vi "Script MessageName.vi"(4 "Message Paths":T5, 6 "Message":T1, 7 "App":refnum<vi>, 8 "error in (no error)":errorcluster, 11 "LV-Protoc in":refnum<class "LV-Protoc.lvclass">) -> (0 "error out":errorcluster, 3 "LV-Protoc out":refnum<class "LV-Protoc.lvclass">)   [LabVIEW 2020, in "LV-Protoc.lvlib" / "LV-Protoc.lvclass"]
uses:
  LV-Protoc.lvclass
  Message Paths.ctl
  LV-Proto/Message.ctl
  LV-Proto/Field.ctl
  LV-Proto/Type.ctl
  LV-Proto/Proto Type.ctl
  <vilib>/Utility/traverseref.llb/TRef TravTarget.ctl
  LV-Protoc.lvlib
  LV-Proto/LV-Proto.lvlib
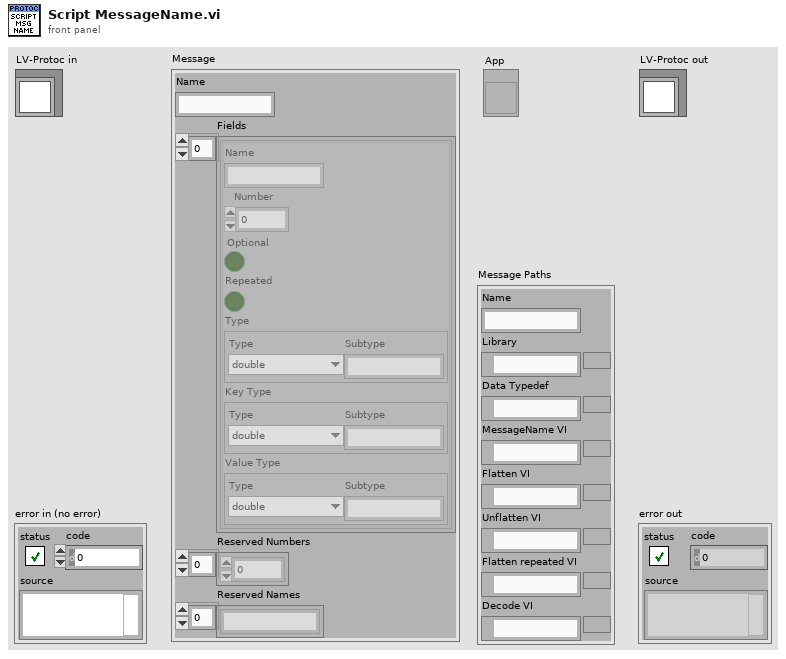
[diagram p1: front panel]
types:
  T1 = typedef "LV-Proto.lvlib/Message.ctl" = cluster{"Name":string, "Fields":T2[], "Reserved Numbers":u32[], "Reserved Names":string[]}
  T2 = typedef "LV-Proto.lvlib/Field.ctl" = cluster{"Name":string, "Number":u32, "Optional":bool, "Repeated":bool, "Type":T3, "Key Type":T3, "Value Type":T3}
  T3 = typedef "LV-Proto.lvlib/Type.ctl" = cluster{"Type":T4, "Subtype":string}
  T4 = typedef "LV-Proto.lvlib/Proto Type.ctl" = enum16{"UNKNOWN", "double", "float", "int32", "int64", "uint32", "uint64", "sint32", "sint64", "fixed32", "fixed64", "sfixed32", "sfixed64", "bool", "string", "bytes", "enum", "map", "message"}
  T5 = typedef "LV-Protoc.lvlib/Message Paths.ctl" = cluster{"Name":string, "Library":path, "Data Typedef":path, "MessageName VI":path, "Flatten VI":path, "Unflatten VI":path, "Flatten repeated VI":path, "Decode VI":path}
  T6 = typedef "TRef TravTarget.ctl" = enum16{"FP", "BD", "Other"}
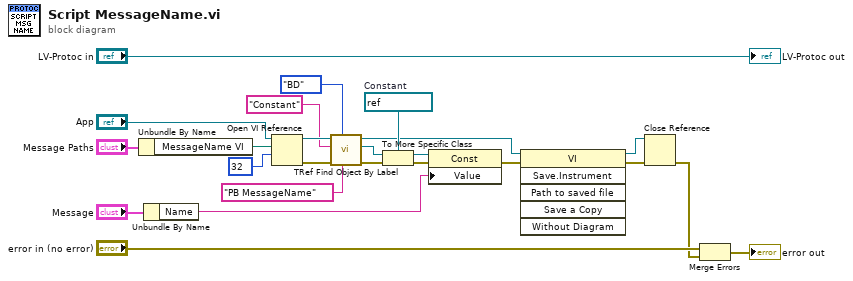
[diagram p0: block diagram]
diagram:
  w11 = refnum<vi> refnum  # Constant
  n1 = Unbundle By Name("Message Paths") -> ("MessageName VI"=w20:path)
  n2 = Unbundle By Name("Message") -> ("Name"=w8:string)
  n3 = Open VI Reference(application reference (local)="App", vi path=w20, options=32) -> (vi reference=w18:refnum<vi>, error out=w17:errorcluster)  [unwired: 3 in]
  n4 = call <vilib>:"TRef Find Object By Label.vi"("Label"="PB MessageName", "Traverse Target"=TRef_TravTarget."BD", "error in (no error)"=w17, "Class Name"="Constant", "VI Ref"=w18) -> ("error out"=w13:errorcluster, "Found Obj Ref"=w12:refnum<vi>, "dup VI Ref"=w5:refnum<vi>)  [unwired: 3 in, 1 out]
  n5 = To More Specific Class(target class=w11, reference=w12, error in=w13) -> (specific class reference=w9:refnum<vi>, error out=w10:errorcluster)
  n6 = property class="Const"(reference=w9, error in=w10, "Value"=w8) -> (error out=w6:errorcluster)  [unwired: 1 out]
  n7 = invoke class="VI" method="Save.Instrument"(reference=w5, error in=w6) -> (reference out=w3:refnum<vi>, error out=w4:errorcluster)  [unwired: 4 in, 4 out]
  n8 = Close Reference(reference=w3, error in (no error)=w4) -> (error out=w2:errorcluster)
  n9 = Merge Errors("error in (no error)", w2) -> (→"error out":errorcluster)
  "LV-Protoc out" <- "LV-Protoc in"
